vi "FABR-Enqueue Run Action.vi"(0 "Run queue":refnum<queue>, 2 "Action":string, 5 "path":path, 7 "Params":T1 {"Sequence"."Level"."Start (dB)" step=5; "Response"."Window (ms)" format="%.2f"}, 9 "Threshold Estimation":T6, 11 "error":errorcluster) -> (4 "queue out":refnum<queue>)   [LabVIEW 2020]
uses:
  Typedefs/FABR-Queue Data.ctl
  Typedefs/FABR-Parameters.ctl
  Typedefs/FABR-Stimulus.ctl
  Typedefs/FABR-Sequence.ctl
  Typedefs/FABR-Order.ctl
  Typedefs/FABR-Response.ctl
  Threshold Estimation VIs/ABR3-Threshold Estimation Parameters.ctl
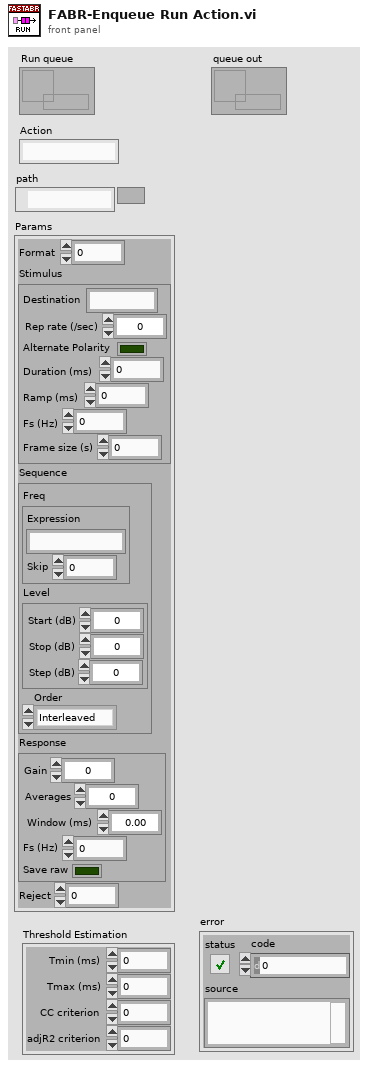
[diagram p1: front panel]
types:
  T1 = typedef "FABR-Parameters.ctl" = cluster{"Format":i32, "Stimulus":T2, "Sequence":T3, "Response":T5, "Reject":dbl}
  T2 = typedef "FABR-Stimulus.ctl" = cluster{"Destination":string, "Rep rate (/sec)":dbl, "Alternate Polarity":bool, "Duration (ms)":dbl, "Ramp (ms)":dbl, "Fs (Hz)":dbl, "Frame size (s)":dbl}
  T3 = typedef "FABR-Sequence.ctl" = cluster{"Freq":cluster{"Expression":string, "Skip":i32}, "Level":cluster{"Start (dB)":i32, "Stop (dB)":i32, "Step (dB)":i32}, "Order":T4}
  T4 = typedef "FABR-Order.ctl" = enum16{"Interleaved", "Step level"}
  T5 = typedef "FABR-Response.ctl" = cluster{"Gain":dbl, "Averages":i32, "Window (ms)":sgl, "Fs (Hz)":dbl, "Save raw":bool}
  T6 = typedef "ABR3-Threshold Estimation Parameters.ctl" = cluster{"Tmin (ms)":dbl, "Tmax (ms)":dbl, "CC criterion":dbl, "adjR2 criterion":dbl}
  T7 = cluster{"Action":string, "path":path, "Params":T1, "Threshold Estimation":T6, "error":errorcluster}
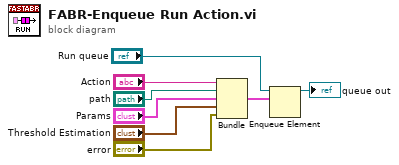
[diagram p0: block diagram]
diagram:
  n1 = Bundle("Action"="Action", "path"="path", "Params"="Params", "Threshold Estimation"="Threshold Estimation", "error"="error") -> (w3:T7)  [unwired: 1 in]
  n2 = Enqueue Element(queue="Run queue", element=w3) -> (queue out=→"queue out":refnum<queue>)  [unwired: 2 in, 2 out]
